vi "fgv_pid_cfg-var.vi"(7 "cmd":T2, 8 "error in":errorcluster, 9 "pid dt":u32, 10 "PID gains":T1={"proportional gain (Kc)"=0.01, "integral time (Ti, min)"=0.0, "derivative time (Td, min)"=0.0} caption="PID gain in" {"derivative time (Td, min)" format="%.6f"; "integral time (Ti, min)" format="%.6f"; "proportional gain (Kc)" format="%.6f"}, 11 "output range":cluster{"output high":dbl, "output low":dbl}={"output high"=0.05, "output low"=-0.05} caption="PID output limit" {"output low" format="%.2f"; "output high" format="%.2f"}) -> (0 "error out":errorcluster, 1 "pid dt out":i64, 2 "PID gains out":T1={"proportional gain (Kc)"=0.01, "integral time (Ti, min)"=0.0, "derivative time (Td, min)"=0.0} caption="PID gain out" {"derivative time (Td, min)" format="%.6f"; "integral time (Ti, min)" format="%.6f"; "proportional gain (Kc)" format="%.6f"}, 3 "output range out":cluster{"output high":dbl, "output low":dbl}={"output high"=0.05, "output low"=-0.05} caption="PID output limit out" {"output low" format="%.2f"; "output high" format="%.2f"})   [LabVIEW 2019]
uses:
  Ctrl/pid-cfg.ctl
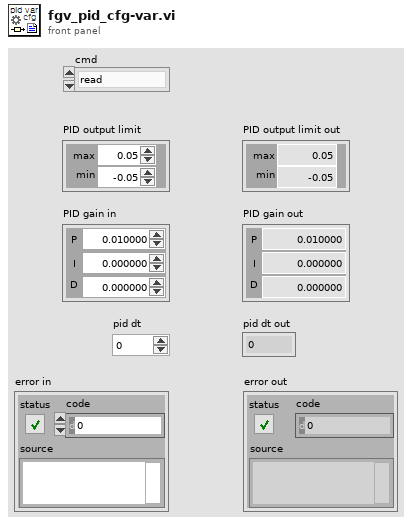
[diagram p1: front panel]
types:
  T1 = cluster{"proportional gain (Kc)":dbl, "integral time (Ti, min)":dbl, "derivative time (Td, min)":dbl}
  T2 = typedef "pid-cfg.ctl" = enum16{"read", "write pid gain", "write pid limit", "pid dt"}
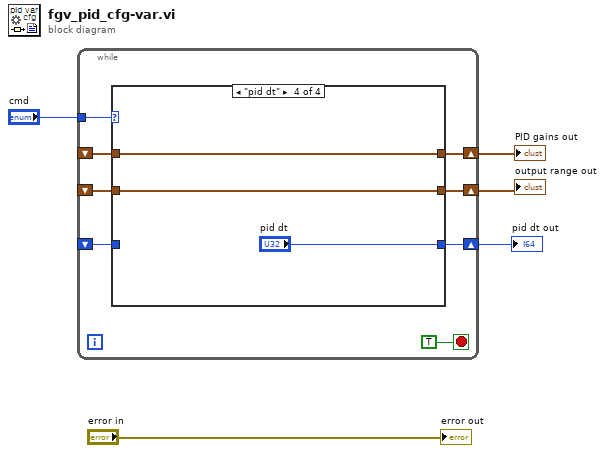
[diagram p0: block diagram]
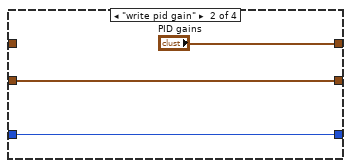
[diagram p3: hidden frame]
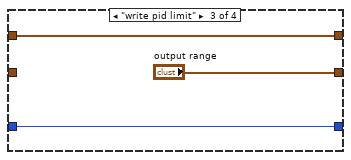
[diagram p4: hidden frame]
diagram:
  n1 = while {
    tunnel: "cmd" -> [w12]
    shift-right: [w11] -> w4
    shift-left: _ -> [w8]
    shift-right: [w10] -> w3
    shift-left: _ -> [w9]
    shift-right: [w7] -> w1
    shift-left: _ -> [w6]
    stop <- TRUE stop-if-true
    n2 = case shown="\"pid dt\"" w12 {
      tunnel: [w16 "PID gains" w21 w25] -> w11
      tunnel: [w15 w18 "output range" w24] -> w10
      tunnel: w9 -> [w15 w18 _ w24]
      tunnel: w8 -> [w16 _ w21 w25]
      tunnel: [w14 w17 w20 "pid dt"] -> w7
      tunnel: w6 -> [w14 w17 w20 _]
      frame "read", Default {
      }
      frame "write pid gain" {
      }
      frame "write pid limit" {
      }
      frame "pid dt" {
      }
    }
  }
  "output range out" <- w3
  "PID gains out" <- w4
  "pid dt out" <- w1
  "error out" <- "error in"
